vi "Assign DUT SIM Slot Profile.vi"(7 "SIM Profile (\"SIMProfile1\")":string="SIMProfile1", 8 "error in (no error)":errorcluster, 9 "SIM Slot (1)":i32=1, 10 "DUT (\"DUT1\")":string="DUT1", 11 "VISA resource name":refnum<visa-resource-name>) -> (0 "error out":errorcluster, 3 "VISA resource name out":refnum<visa-resource-name>)   [LabVIEW 2020, in "Rohde&Schwarz CMXP Base.lvlib"]
doc: "Assigns the SIM profile to the SlM slot number of the inactive DUT.\n\nAttribute:\nRSCMXPBASE_ATTR_SELECT_DUT_SIM_SLOT\n\nRemote-control command:\n[CONFigure:]DUT:PROFile:SIMSlot<no>:SIMProfile"
uses:
  <instrlib>/Rohde&Schwarz CMXP Base/Rohde&Schwarz CMXP Base.lvlib
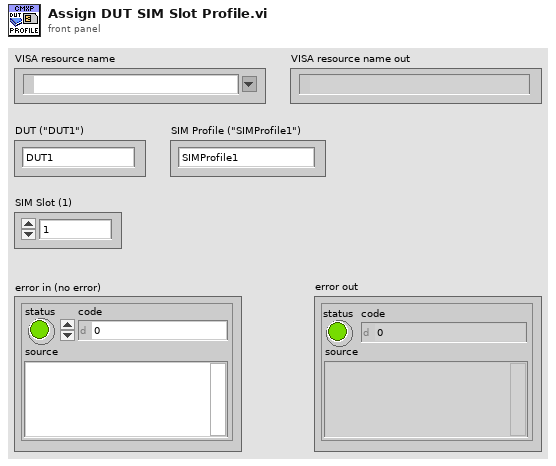
[diagram p1: front panel]
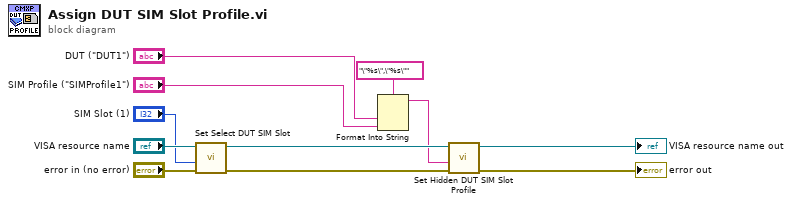
[diagram p0: block diagram]
diagram:
  n1 = call "Set Select DUT SIM Slot"("error in (no error)"="error in (no error)", "Select DUT SIM Slot (0)"="SIM Slot (1)", "instrument handle"="VISA resource name") -> ("error out"=w3:errorcluster, "instrument handle out"=w5:refnum<visa-resource-name>)  [unwired: 7 in]
  n2 = Format Into String(format string="\"%s\",\"%s\"", "DUT (\"DUT1\")", "SIM Profile (\"SIMProfile1\")") -> (resulting string=w2:string)  [unwired: 2 in, 1 out]
  n3 = call "Set Hidden DUT SIM Slot Profile"("error in (no error)"=w3, "Hidden DUT SIM Slot Profile ()"=w2, "instrument handle"=w5) -> ("error out"=→"error out":errorcluster, "instrument handle out"=→"VISA resource name out":refnum<visa-resource-name>)  [unwired: 7 in]
